vi "Change timing to seconds.vi"(8 "error in (no error)":errorcluster, 10 "Time (sec)":dbl=1.0, 11 "Elevator Controller Actor in":refnum<class "Elevator Controller Actor.lvclass">) -> (0 "error out":errorcluster, 3 "Elevator Controller Actor out":refnum<class "Elevator Controller Actor.lvclass">)   [LabVIEW 2019, in "Elevator Controller Actor.lvlib" / "Elevator Controller Actor.lvclass"]
uses:
  Elevator Controller Actor.lvclass
  Sim Display Console Actor/Sim Display Console Actor Messages/Write Timing Msg/Write Timing Msg.lvclass
  Elevator Controller Actor Messages/Set Enable Door Msg/Set Enable Door Msg.lvclass
  <vilib>/ActorFramework/Actor/Actor.lvclass
  Sim User Console Actor/Elevator Controller/Floor Selection.ctl
  Sim User Console Actor/Elevator Controller/Sim User Console Actor.lvclass
  Sim User Console Actor/Sim User Console Actor Messages/Write Floor Selection Msg/Write Floor Selection Msg.lvclass
  C:/Program Files (x86)/National Instruments/LabVIEW 2019/vi.lib/ActorFramework/Actor/Actor.lvclass
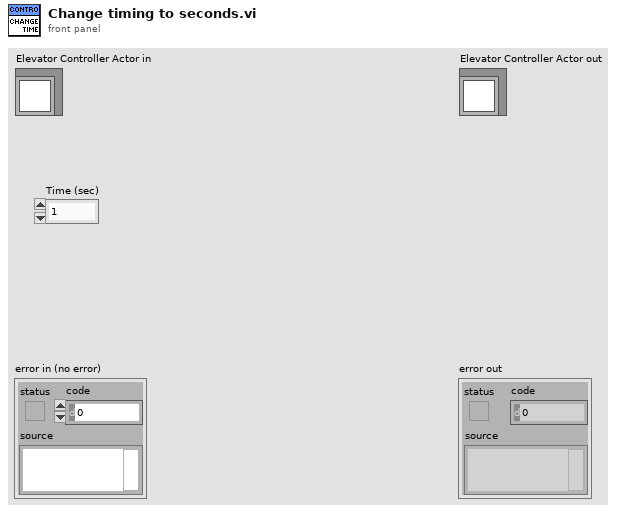
[diagram p1: front panel]
types:
  T1 = enum8{"Enabled", "Disabled", "Disabled and Grayed Out"}
  T2 = typedef "Simulated User Console Actor.lvlib/Sim User Console Actor.lvclass/Floor Selection.ctl" = cluster{"Floor4":bool, "Floor 3":bool, "Floor2":bool, "Floor1":bool}
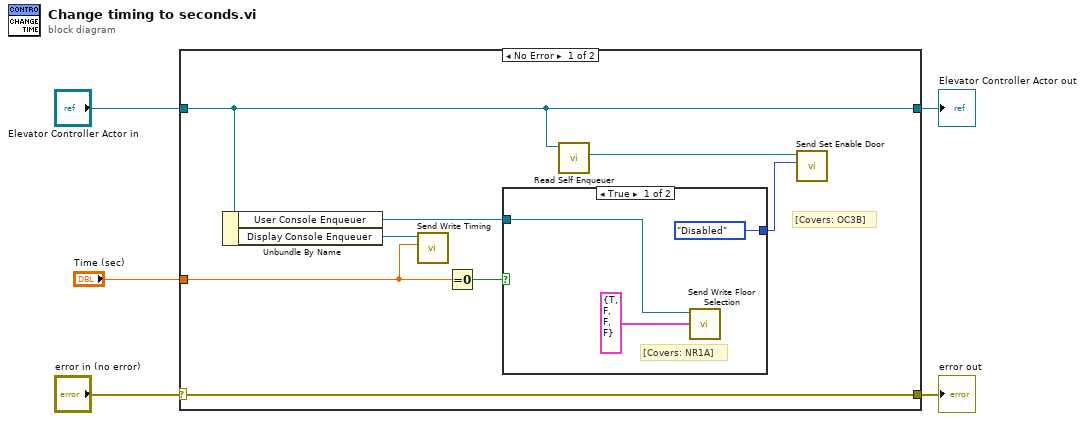
[diagram p0: block diagram]
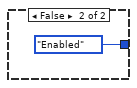
[diagram p2: hidden frame]
diagram:
  n1 = case shown="No Error" "error in (no error)" {
    selector: "error in (no error)" -> [w13 w19]
    tunnel: [w13 w19] -> w4
    tunnel: [w10 w18] -> w2
    tunnel: "Elevator Controller Actor in" -> [w10 w18]
    tunnel: "Time (sec)" -> [w11 _]
    frame No Error {
      # "[Covers: OC3B]"
      n2 = Unbundle By Name(w10) -> ("User Console Enqueuer"=w6:refnum<class "Message Enqueuer.lvclass">, "Display Console Enqueuer"=w12:refnum<class "Message Enqueuer.lvclass">)
      n3 = call "Send Write Timing.vi"("Time"=w11, "Message Enqueuer"=w12) -> ()  [unwired: 8 in, 2 out]
      n4 = Equal To 0?(x=w11) -> (x = 0?=w9:bool)
      n5 = case shown="True" w9 {
        tunnel: [T1."Disabled" ("Disabled") T1."Enabled" ("Disabled")] -> w7
        tunnel: w6 -> [w15 _]
        frame True {
          # "[Covers: NR1A]"
          n6 = call "Send Write Floor Selection.vi"("Floor Selection"=T2 {"Floor4"=TRUE, "Floor 3"=FALSE, "Floor2"=FALSE, "Floor1"=FALSE} ("Value"), "Message Enqueuer"=w15) -> ()  [unwired: 8 in, 2 out]
        }
        frame False {
        }
      }
      n7 = call <vilib>:"Read Self Enqueuer.vi"("Actor"=w10) -> ("Self Enqueuer"=w8:refnum<class "Message Enqueuer.lvclass">)  [unwired: 10 in]
      n8 = call "Send Set Enable Door.vi"("Disabled"=w7, "Message Enqueuer"=w8) -> ()  [unwired: 8 in, 2 out]
    }
    frame Error {
    }
  }
  "error out" <- w4
  "Elevator Controller Actor out" <- w2
